vi "loadPeelData.vi"(10 "path":path=path "C:/M300/peel") -> ()   [LabVIEW 2012]
uses:
  <vilib>/Utility/NIReport.llb/NI_report.lvclass
  <vilib>/addons/database/Connection.llb/DB Tools Open Connec (Path).vi
  <vilib>/addons/database/Connection.llb/Conn Execute.vi
  <vilib>/addons/database/Recordset.llb/Rec Destroy - Connection.vi
  <vilib>/Utility/NIReport.llb/Excel/NI_Excel.lvclass
  <vilib>/addons/database/NI_Database_API.lvlib
panel:
  out "error out":errorcluster
  out "data":string
  out "filenames":string[](array[string])
  out "error out 4":errorcluster
  in  "Cluster":T1
  out "after substring":string
  out "data 3":string
  out "data 15":string
  out "data 14":string
  out "data 13":string
  out "data 12":string
  out "data 11":string
  out "data 10":string
  out "data 9":string
  out "data 8":string
  out "data 7":string
  out "data 6":string
  out "data 5":string
  out "data 4":string
  out "data 2":string
  out "OP":string
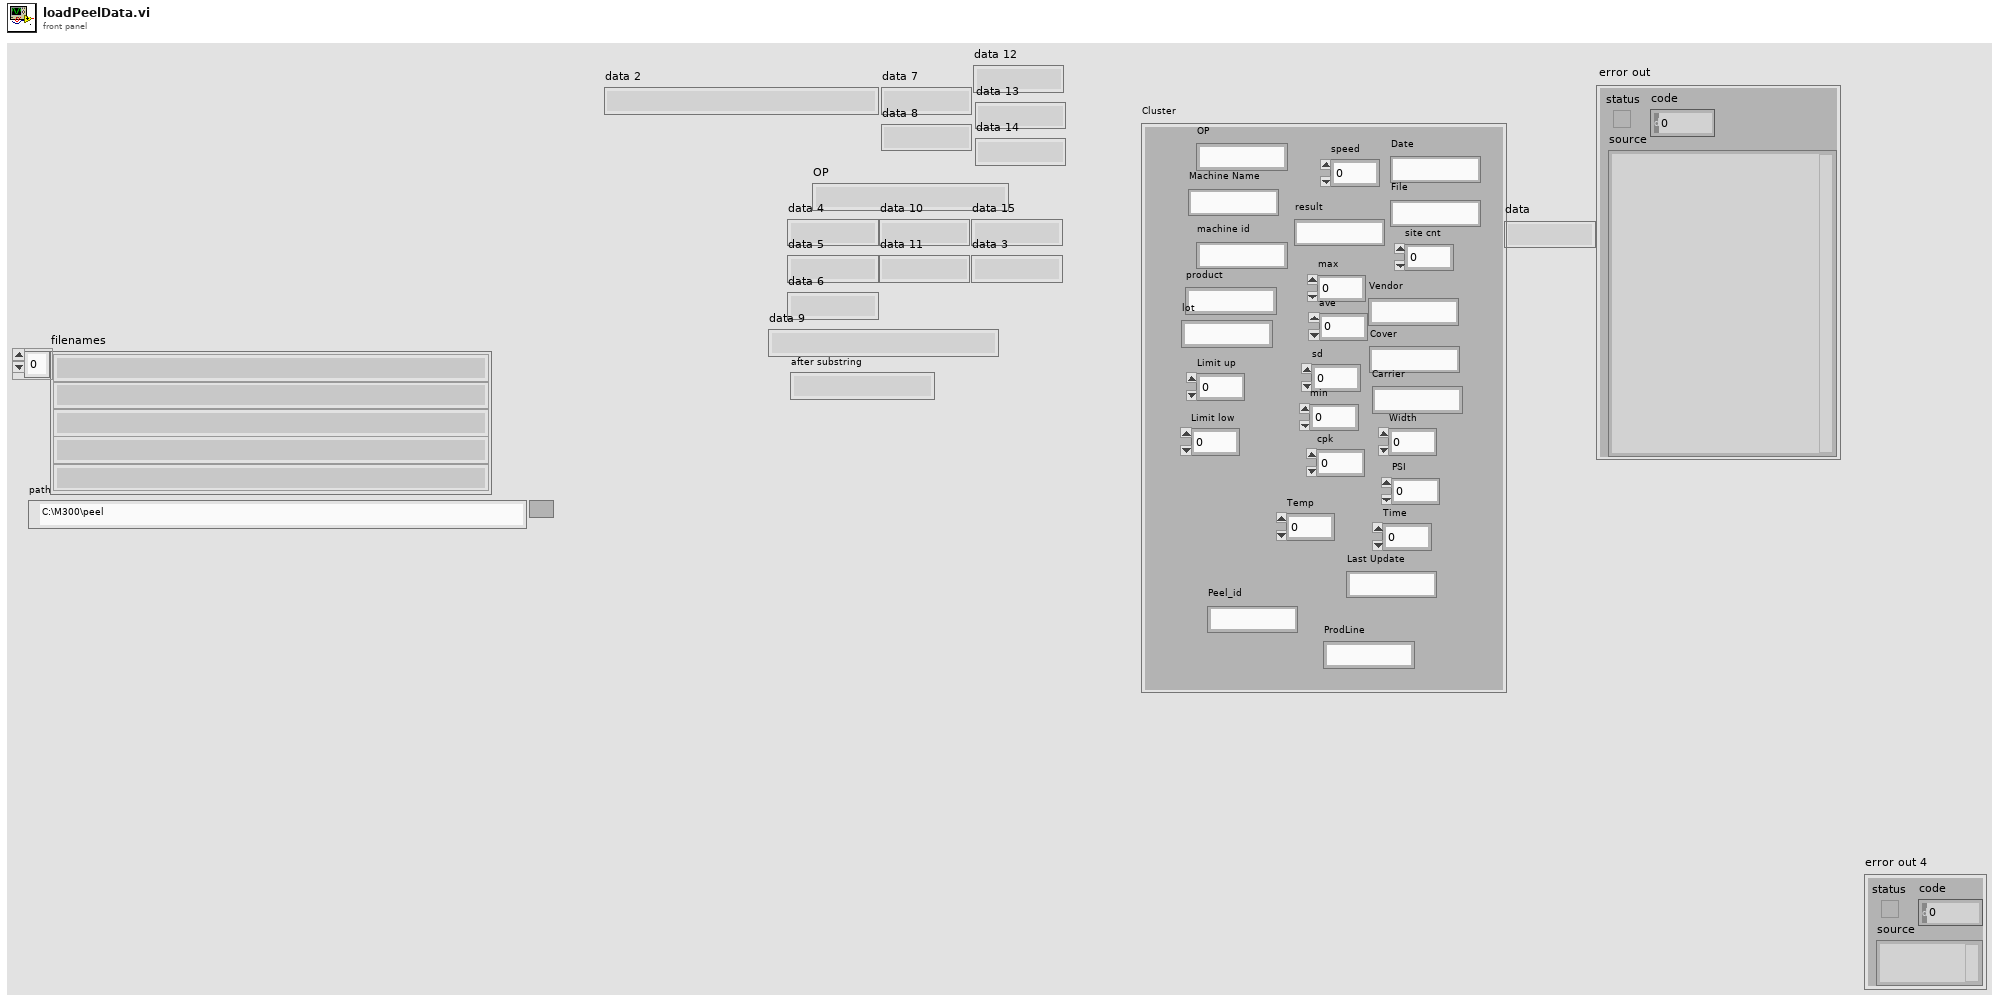
[diagram p1: front panel]
types:
  T1 = cluster{"OP":string, "Machine Name ":string, "machine id ":string, "product ":string, "lot":string, "Limit up":dbl, "Limit low":dbl, "speed":dbl, "result ":string, "max":dbl, "ave":dbl, "sd ":dbl, "min":dbl, "cpk":dbl, "Date ":string, "File ":string, "site cnt":dbl, "Vendor":string, "Cover":string, "Carrier":string, "Width":dbl, "PSI":dbl, "Temp":dbl, "Time":dbl, "Last Update":string, "Peel_id":string, "ProdLine":string}
  T2 = typedef "NI_Database_API.lvlib/Conn ObjectReference.ctl" = refnum<k1>
  T3 = enum16{"Standard Report", "HTML", "Word", "Excel"}
  T4 = typedef "NI_Database_API.lvlib/Rec ObjectReference.ctl" = refnum<k1>
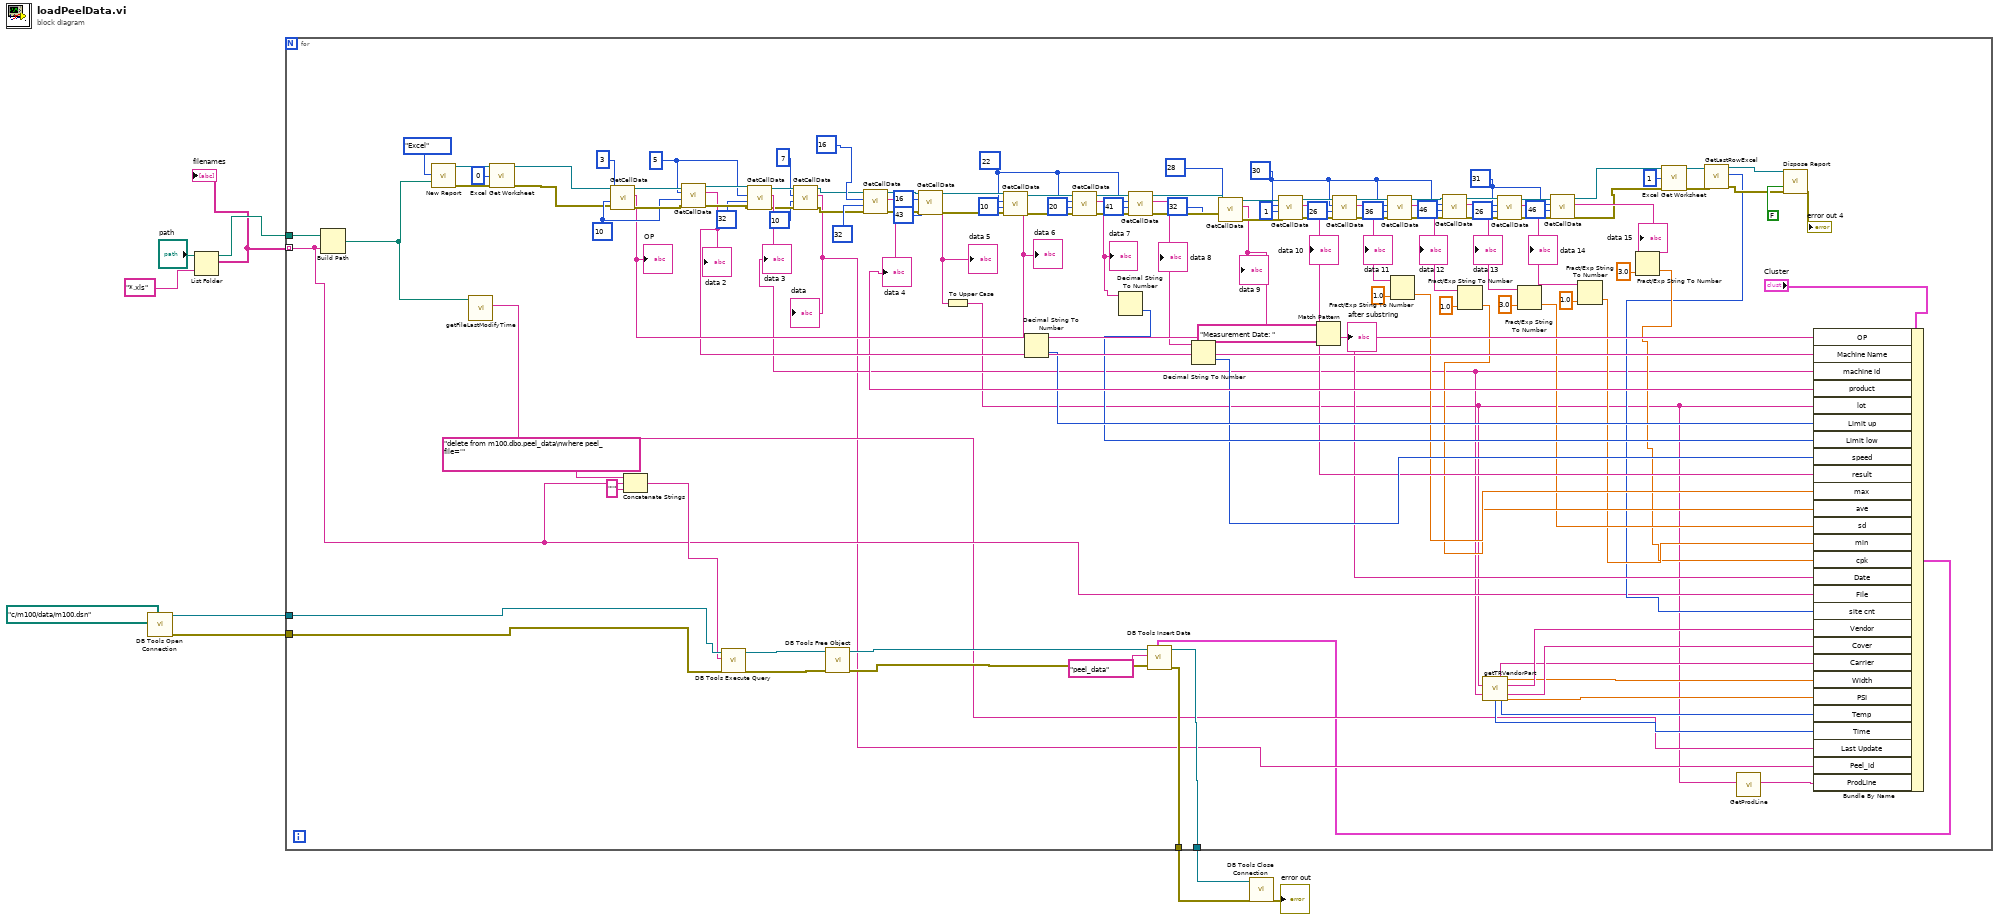
[diagram p0: block diagram]
diagram:
  n1 = call-poly <vilib>:"DB Tools Open Connection.vi"("connection information"=path "c:/m100/data/m100.dsn") -> ("error out"=w4:errorcluster, "connection reference"=w5:T2)  [unwired: 7 in]
  n2 = List Folder(path="path", pattern="*.xls") -> (path out=w8:path, filenames=w7:string[])  [unwired: 2 in, 2 out]
  "filenames" <- w7
  n3 = for {
    tunnel: w8 -> [w54]
    tunnel: w7 -> [w36] mode=indexing
    tunnel: w5 -> [w51]
    tunnel: w4 -> [w50]
    tunnel: [w53] -> w3
    tunnel: [w52] -> w2
    w97 = 31 ("start row")
    w105 = 30 ("start row")
    w123 = 22 ("start row")
    w89 = 5 ("start row")
    w91 = 10 ("start column")
    n4 = Build Path(base path=w54, name or relative path=w36) -> (appended path=w24:path)
    n5 = call <vilib>:"New Report.vi"("report type"=T3."Excel" ("Report Type"), "template (empty)"=w24) -> ("report out"=w137:refnum<class "NI_report.lvclass">, "error out"=w136:errorcluster)  [unwired: 12 in]
    n6 = call "getFileLastModifyTime.vi"("path"=w24) -> ("date/time string"=w23:string)  [unwired: 10 in]
    n7 = call <vilib>:"Excel Get Worksheet.vi"("report in"=w137, "worksheet index (0)"=0, "error in (no error)"=w136) -> ("report out"=w56:refnum<class "NI_report.lvclass">, "error out"=w55:errorcluster)  [unwired: 11 in]
    n8 = call "GetCellData.vi"("error in (no error)"=w55, "start column"=w91, "start row"=3, "report in"=w56) -> ("error out"=w94:errorcluster, "data"=w84:string, "report out"=w95:refnum<class "NI_report.lvclass">)  [unwired: 5 in]
    "OP" <- w84
    n9 = Concatenate Strings("delete from m100.dbo.peel_data\nwhere peel_file='" ("string"), w36, "'" ("string")) -> (w46:string)
    n10 = call "GetCellData.vi"("error in (no error)"=w94, "start column"=w91, "start row"=w89, "report in"=w95) -> ("error out"=w93:errorcluster, "data"=w83:string, "report out"=w90:refnum<class "NI_report.lvclass">)  [unwired: 5 in]
    "data 2" <- w83
    n11 = call-poly <vilib>:"DB Tools Execute Query.vi"("error in (no error)"=w50, "SQL query"=w46, "connection reference"=w51) -> ("error out"=w25:errorcluster, "recordset reference"=w26:T4)  [unwired: 5 in]
    n12 = call "GetCellData.vi"("error in (no error)"=w93, "start column"=32, "start row"=w89, "report in"=w90) -> ("error out"=w22:errorcluster, "data"=w35:string, "report out"=w21:refnum<class "NI_report.lvclass">)  [unwired: 5 in]
    "data 3" <- w35
    n13 = call "GetCellData.vi"("error in (no error)"=w22, "start column"=10, "start row"=7, "report in"=w21) -> ("error out"=w18:errorcluster, "data"=w15:string, "report out"=w19:refnum<class "NI_report.lvclass">)  [unwired: 5 in]
    "data" <- w15
    n14 = call-poly <vilib>:"DB Tools Free Object.vi"("error in (no error)"=w25, "recordset reference"=w26) -> ("error out"=w49:errorcluster, "connection reference"=w48:T2)  [unwired: 8 in]
    n15 = call "GetCellData.vi"("error in (no error)"=w18, "start column"=32, "start row"=16, "report in"=w19) -> ("error out"=w132:errorcluster, "data"=w82:string, "report out"=w133:refnum<class "NI_report.lvclass">)  [unwired: 5 in]
    "data 4" <- w82
    n16 = call "GetCellData.vi"("error in (no error)"=w132, "start column"=43, "start row"=16, "report in"=w133) -> ("error out"=w125:errorcluster, "data"=w12:string, "report out"=w126:refnum<class "NI_report.lvclass">)  [unwired: 5 in]
    "data 5" <- w12
    n17 = To Upper Case(1:w12) -> (0:w11:string)
    n18 = call "GetCellData.vi"("error in (no error)"=w125, "start column"=10, "start row"=w123, "report in"=w126) -> ("error out"=w128:errorcluster, "data"=w81:string, "report out"=w129:refnum<class "NI_report.lvclass">)  [unwired: 5 in]
    "data 6" <- w81
    n19 = Decimal String To Number(string=w81) -> (number=w80:i32)  [unwired: 2 in, 1 out]
    n20 = call "GetCellData.vi"("error in (no error)"=w128, "start column"=20, "start row"=w123, "report in"=w129) -> ("error out"=w127:errorcluster, "data"=w79:string, "report out"=w124:refnum<class "NI_report.lvclass">)  [unwired: 5 in]
    "data 7" <- w79
    n21 = Decimal String To Number(string=w79) -> (number=w78:i32)  [unwired: 2 in, 1 out]
    n22 = call "GetCellData.vi"("error in (no error)"=w127, "start column"=41, "start row"=w123, "report in"=w124) -> ("error out"=w118:errorcluster, "data"=w77:string, "report out"=w119:refnum<class "NI_report.lvclass">)  [unwired: 5 in]
    "data 8" <- w77
    n23 = Decimal String To Number(string=w77) -> (number=w76:i32)  [unwired: 2 in, 1 out]
    n24 = call "GetCellData.vi"("error in (no error)"=w118, "start column"=32, "start row"=28, "report in"=w119) -> ("error out"=w111:errorcluster, "data"=w87:string, "report out"=w115:refnum<class "NI_report.lvclass">)  [unwired: 5 in]
    "data 9" <- w87
    n25 = call "GetCellData.vi"("error in (no error)"=w111, "start column"=1, "start row"=w105, "report in"=w115) -> ("error out"=w110:errorcluster, "data"=w75:string, "report out"=w114:refnum<class "NI_report.lvclass">)  [unwired: 5 in]
    "data 10" <- w75
    n26 = Match Pattern(string=w87, regular expression="Measurement Date: ") -> (after substring=w59:string)  [unwired: 1 in, 3 out]
    "after substring" <- w59
    n27 = call "GetCellData.vi"("error in (no error)"=w110, "start column"=26, "start row"=w105, "report in"=w114) -> ("error out"=w109:errorcluster, "data"=w74:string, "report out"=w113:refnum<class "NI_report.lvclass">)  [unwired: 5 in]
    "data 11" <- w74
    n28 = call "GetCellData.vi"("error in (no error)"=w109, "start column"=36, "start row"=w105, "report in"=w113) -> ("error out"=w108:errorcluster, "data"=w71:string, "report out"=w106:refnum<class "NI_report.lvclass">)  [unwired: 5 in]
    "data 12" <- w71
    n29 = Fract/Exp String To Number(string=w74, default (0 dbl)=1.0 ("default (0 DBL)")) -> (number=w72:dbl)  [unwired: 2 in, 1 out]
    n30 = call "GetCellData.vi"("error in (no error)"=w108, "start column"=46, "start row"=w105, "report in"=w106) -> ("error out"=w107:errorcluster, "data"=w68:string, "report out"=w112:refnum<class "NI_report.lvclass">)  [unwired: 5 in]
    "data 13" <- w68
    n31 = Fract/Exp String To Number(string=w71, default (0 dbl)=1.0 ("default (0 DBL)")) -> (number=w69:dbl)  [unwired: 2 in, 1 out]
    n32 = call "getTRVendorPart.vi"("RC No"=w11, "Machine"=w35) -> ("Carrier"=w32:string, "Width"=w31:dbl, "Vendor"=w34:string, "Cover"=w33:string, "Time"=w28:i32, "Temp"=w29:i32, "PSI"=w30:dbl)  [unwired: 7 in]
    n33 = call "GetCellData.vi"("error in (no error)"=w107, "start column"=26, "start row"=w97, "report in"=w112) -> ("error out"=w98:errorcluster, "data"=w65:string, "report out"=w99:refnum<class "NI_report.lvclass">)  [unwired: 5 in]
    "data 14" <- w65
    n34 = Fract/Exp String To Number(string=w68, default (0 dbl)=3.0 ("default (0 DBL)")) -> (number=w66:dbl)  [unwired: 2 in, 1 out]
    n35 = call "GetCellData.vi"("error in (no error)"=w98, "start column"=46, "start row"=w97, "report in"=w99) -> ("error out"=w43:errorcluster, "data"=w62:string, "report out"=w44:refnum<class "NI_report.lvclass">)  [unwired: 5 in]
    "data 15" <- w62
    n36 = Fract/Exp String To Number(string=w65, default (0 dbl)=1.0 ("default (0 DBL)")) -> (number=w63:dbl)  [unwired: 2 in, 1 out]
    n37 = Fract/Exp String To Number(string=w62, default (0 dbl)=3.0 ("default (0 DBL)")) -> (number=w60:dbl)  [unwired: 2 in, 1 out]
    n38 = call <vilib>:"Excel Get Worksheet.vi"("report in"=w44, "worksheet index (0)"=1, "error in (no error)"=w43) -> ("report out"=w41:refnum<class "NI_report.lvclass">, "error out"=w39:errorcluster)  [unwired: 11 in]
    n39 = call "GetLastRowExcel.vi"("error in (no error)"=w39, "report in"=w41) -> ("error out"=w38:errorcluster, "row"=w37:i32, "report out"=w40:refnum<class "NI_report.lvclass">)  [unwired: 7 in]
    n40 = call "GetProdLine.vi"("Lotno"=w11) -> ("ProdLine"=w13:string)  [unwired: 10 in]
    n41 = call-dynamic "Dispose Report.vi"("report in"=w40, "save changes? (F)"=FALSE, "error in (no error)"=w38) -> ("error out"=→"error out 4":errorcluster)  [unwired: 12 in]
    n42 = Bundle By Name(cluster="Cluster", "OP"=w84, "Machine Name"=w83, "machine id"=w35, "product"=w82, "lot"=w11, "Limit up"=w80, "Limit low"=w78, "speed"=w76, "result"=w75, "max"=w72, "ave"=w69, "sd"=w66, "min"=w63, "cpk"=w60, "Date"=w59, "File"=w36, "site cnt"=w37, "Vendor"=w34, "Cover"=w33, "Carrier"=w32, "Width"=w31, "PSI"=w30, "Temp"=w29, "Time"=w28, "Last Update"=w23, "Peel_id"=w15, "ProdLine"=w13) -> (w14:T1)
    n43 = call <vilib>:"DB Tools Insert Data.vi"("data"=w14, "error in (no error)"=w49, "table"="peel_data", "connection reference"=w48) -> ("error out"=w52:errorcluster, "connection reference out"=w53:T2)  [unwired: 6 in]
  }
  n44 = call <vilib>:"DB Tools Close Connection.vi"("error in (no error)"=w2, "connection reference"=w3) -> ("error out"=→"error out":errorcluster)  [unwired: 5 in]
